vi "Test Change Handler Log Level.vi"(8 "error in":errorcluster) -> (0 "error out":errorcluster)   [LabVIEW 2016, in "UT_Helper.lvlib"]
doc: "Test if there is no error after an existent Logger was closed.\nTest if there is an error after the close was called again."
uses:
  UT_Helper.lvlib
  Source/HSE-Logger/Handler/Handler.lvclass
  Source/HSE-Logger/LogLevel.ctl
  <vilib>/addons/_JKI Toolkits/Caraya/classes/Assert/Assert Equal Value_Variant.vi
  Source/HSE-Logger/hse-logger.lvlib
  <vilib>/addons/_JKI Toolkits/Caraya/classes/Test/Test.lvclass
  <vilib>/addons/_JKI Toolkits/Caraya/classes/Assert/Assert.lvclass
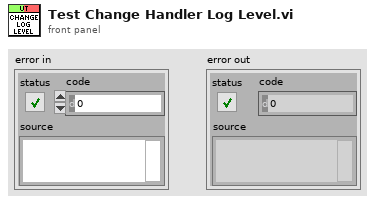
[diagram p1: front panel]
types:
  T1 = typedef "hse-logger.lvlib/LogLevel.ctl" = enum16{"DEBUG", "INFO", "WARNING", "ERROR", "CRITICAL"}
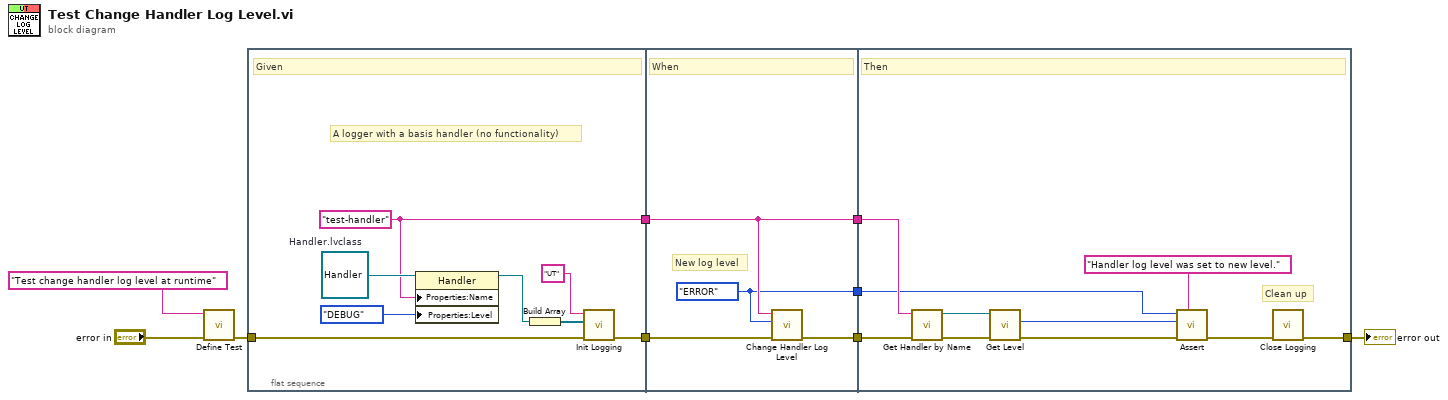
[diagram p0: block diagram]
diagram:
  n1 = call <vilib>:"Define Test.vi"("error in (no error)"="error in", "Label (VI Title)"="Test change handler log level at runtime") -> ("error out"=w5:errorcluster)  [unwired: 8 in, 1 out]
  n2 = flat-sequence {
    tunnel: w5 -> [w11]
    tunnel: [w17] -> w9
    tunnel: [w10] -> w3
    tunnel: w9 -> [w21]
    tunnel: [w20] -> w8
    tunnel: w3 -> [w19]
    tunnel: [w19] -> w2
    tunnel: [w18] -> w1
    tunnel: [w22] -> w7
    tunnel: w8 -> [w31]
    tunnel: w2 -> [w30]
    tunnel: w1 -> [w24]
    frame #0 {
      w10 = "test-handler" ("Name")
      w14 = refnum<class "Handler.lvclass"> refnum  # Handler.lvclass
      # "A logger with a basis handler (no functionality)"
      # "Given"
      n3 = property class="Handler"(reference=w14, "Properties:Name"=w10, "Properties:Level"=LogLevel."DEBUG" ("Level")) -> (reference out=w13:refnum<class "Handler.lvclass">)  [unwired: 1 in, 1 out]
      n4 = Build Array(w13) -> (w15:refnum<class "Handler.lvclass">[])
      n5 = call "Init Logging.vi"("error in"=w11, "Handlers"=w15, "Name"="UT") -> ("error out"=w17:errorcluster)  [unwired: 8 in]
    }
    frame #1 {
      w18 = LogLevel."ERROR" ("New Log Level")
      # "New log level"
      # "When"
      n6 = call "Change Handler Log Level.vi"("error in"=w21, "New Log Level"=w18, "Handler Name"=w19) -> ("error out"=w20:errorcluster)  [unwired: 8 in]
    }
    frame #2 {
      # "Clean up"
      # "Then"
      n7 = call "Get Handler by Name.vi"("error in"=w31, "Name"=w30) -> ("error out"=w29:errorcluster, "Handler out"=w28:refnum<class "Handler.lvclass">)  [unwired: 8 in]
      n8 = call-dynamic "Get Level.vi"("error in"=w29, "Handler in"=w28) -> ("error out"=w27:errorcluster, "Level"=w25:T1)  [unwired: 7 in, 1 out]
      n9 = call-poly <vilib>:"Assert.vi"("Label"="Handler log level was set to new level.", "error in (no error)"=w27, "Y"=w25, "X"=w24) -> ("error out"=w23:errorcluster)  [unwired: 6 in, 1 out]
      n10 = call "Close Logging.vi"("error in"=w23) -> ("error out"=w22:errorcluster)  [unwired: 10 in]
    }
  }
  "error out" <- w7
